vi "Logger Create Date-Time file.vi"(0 "File name":string, 5 "Desired path":string, 11 "error in (no error)":errorcluster) -> (4 "Path and name":path, 15 "error out":errorcluster)   [LabVIEW 2018]
uses:
  Logger Global.vi
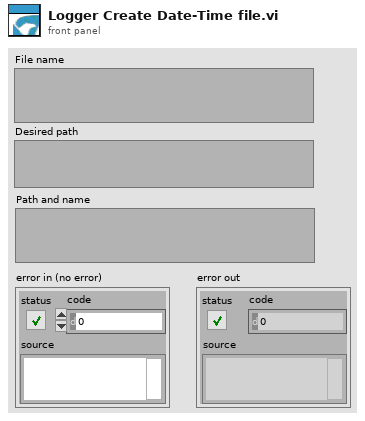
[diagram p1: front panel]
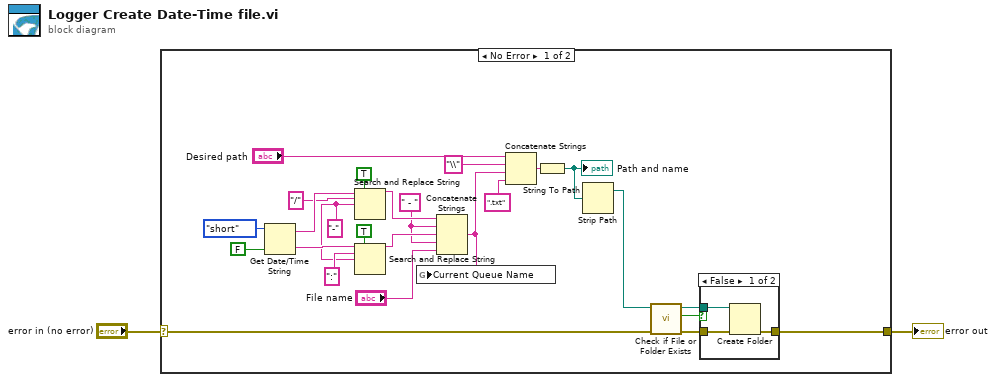
[diagram p0: block diagram]
diagram:
  n1 = case shown="No Error" "error in (no error)" {
    selector: "error in (no error)" -> [w8 w32]
    tunnel: [w9 w32] -> w1
    frame No Error {
      w14 = "-" ("string")
      w19 = " - " ("string")
      n2 = Get Date/Time String(date format (0)=enum16{"short", "long", "abbreviated"}."short", want seconds? (F)=FALSE) -> (date string=w13:string, time string=w16:string)  [unwired: 1 out]
      n3 = Search and Replace String(replace all?=TRUE ("replace all? (F)"), input string=w13, search string="/", replace string=w14) -> (result string=w20:string)  [unwired: 1 in, 6 out]
      n4 = Search and Replace String(replace all?=TRUE ("replace all? (F)"), input string=w16, search string=":", replace string=w14) -> (result string=w21:string)  [unwired: 1 in, 6 out]
      n5 = Concatenate Strings(w20, w19, w21, w19, "File name") -> (w4:string)
      n6 = global write "Logger Global.vi" "Current Queue Name"(w4) -> ()
      n7 = Concatenate Strings("Desired path", "\\" ("search string"), w4, ".txt" ("string")) -> (w7:string)
      n8 = String To Path(string=w7) -> (path=w23:path)
      "Path and name" <- w23
      n9 = Strip Path(path=w23) -> (stripped path=w24:path)  [unwired: 1 out]
      n10 = call <vilib>:"Check if File or Folder Exists.vi"("error in (no error)"=w8, "path"=w24) -> ("error out"=w27:errorcluster, "file or folder exists?"=w26:bool, "dup path"=w25:path)  [unwired: 7 in]
      n11 = case shown="False" w26 {
        tunnel: w25 -> [w30 _]
        tunnel: [w29 w31] -> w9
        tunnel: w27 -> [w28 w31]
        frame False {
          n12 = Create Folder(path (use dialog)=w30, error in=w28) -> (error out=w29:errorcluster)  [unwired: 1 in, 2 out]
        }
        frame True {
        }
      }
    }
    frame Error {
    }
  }
  "error out" <- w1
